vi "Get Mediator Settings.vi"(8 "error in (no error)":errorcluster, 11 "Custom Device Ref in":T2 format="%.0x") -> (0 "error out":errorcluster, 2 "Mediator Settings":T1, 3 "Custom Device Ref out":T2 format="%.0x")   [LabVIEW 2016, in "VeriStand Configuration Support.lvlib"]
uses:
  VeriStand Configuration Support.lvlib
  <vilib>/NI Veristand/Custom Device API/Custom Device Item Ref.ctl
  Mediator Settings.ctl
  Constants.vi
  <vilib>/NI Veristand/Custom Device API/Get Item Property (Variant).vi
  <vilib>/NI Veristand/Custom Device API/Set Item Property (Variant).vi
  <vilib>/NI Veristand/Custom Device API/Custom Device API.lvlib
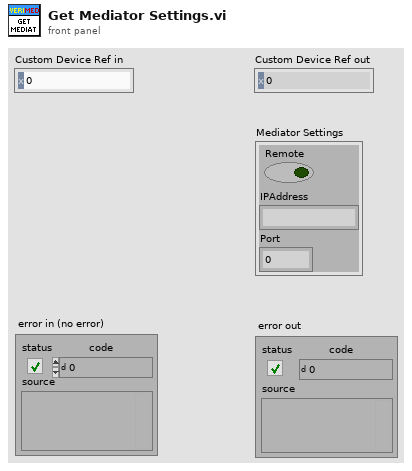
[diagram p1: front panel]
types:
  T1 = typedef "VeriStand Configuration Support.lvlib/Mediator Settings.ctl" = cluster{"Remote":bool, "IPAddress":string, "Port":u16}
  T2 = typedef "Custom Device API.lvlib/Custom Device Item Ref.ctl" = u64
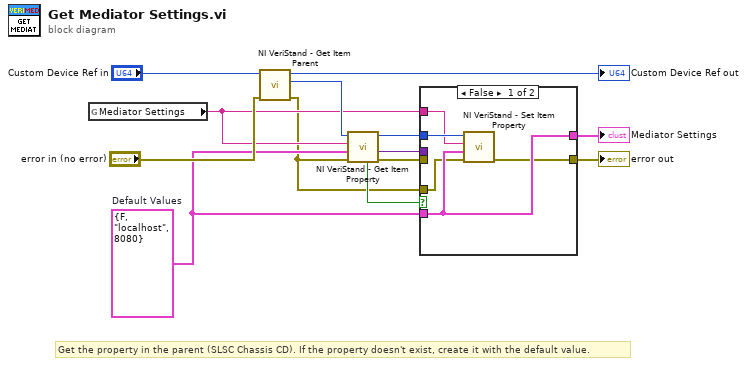
[diagram p0: block diagram]
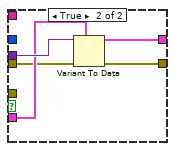
[diagram p2: hidden frame]
diagram:
  w8 = T1 {"Remote"=FALSE, "IPAddress"="localhost", "Port"=8080}  # Default Values
  # "Get the property in the parent (SLSC Chassis CD). If the property doesn't exist, create it with the default value."
  n1 = global read "Constants.vi" "Mediator Settings"() -> (w4:string)
  n2 = call <vilib>:"NI VeriStand - Get Item Parent.vi"("error in (no error)"="error in (no error)", "Item Ref in"="Custom Device Ref in") -> ("error out"=w1:errorcluster, "Parent Ref"=w10:T2, "Item Ref out"=→"Custom Device Ref out":T2)  [unwired: 6 in, 1 out]
  n3 = call-poly <vilib>:"NI VeriStand - Get Item Property.vi"("error in (no error)"=w1, "Default Value"=w8, "Property Name"=w4, "Item Ref in"=w10) -> ("error out"=w2:errorcluster, "Value"=w9:variant, "Item Ref out"=w5:T2, "Found?"=w3:bool)  [unwired: 4 in]
  n4 = case shown="False" w3 {
    tunnel: w9 -> [_ w23]
    tunnel: w8 -> [w16 w22]
    tunnel: [w15 w21] -> w6
    tunnel: [w16 w20] -> w7
    tunnel: w5 -> [w18 _]
    tunnel: w4 -> [w17 _]
    tunnel: w2 -> [_ w19]
    tunnel: w1 -> [w14 _]
    frame False {
      n5 = call-poly <vilib>:"NI VeriStand - Set Item Property.vi"("error in (no error)"=w14, "Value"=w16, "Property Name"=w17, "Item Ref in"=w18) -> ("error out"=w15:errorcluster)  [unwired: 5 in, 2 out]
    }
    frame True {
      n6 = Variant To Data(error in=w19, type=w22, Variant=w23) -> (data=w20:T1, error out=w21:errorcluster)
    }
  }
  "error out" <- w6
  "Mediator Settings" <- w7
